vi "ReadWrite.ProcessData.vi"(8 "error in (no error)":errorcluster, 10 "timeout ms":i32=100, 11 "ReadWrite in":refnum<class "ReadWrite.lvclass">) -> (0 "error out":errorcluster, 1 "Timeout?":bool, 2 "Values":dbl[](array[numeric]), 3 "ReadWrite out":refnum<class "ReadWrite.lvclass">)   [LabVIEW 2015, in "Data Access Engine.lvlib" / "ReadWrite.lvclass"]
uses:
  ReadWrite.lvclass
  ReadWrite.lvclass/ReadWrite.ctl
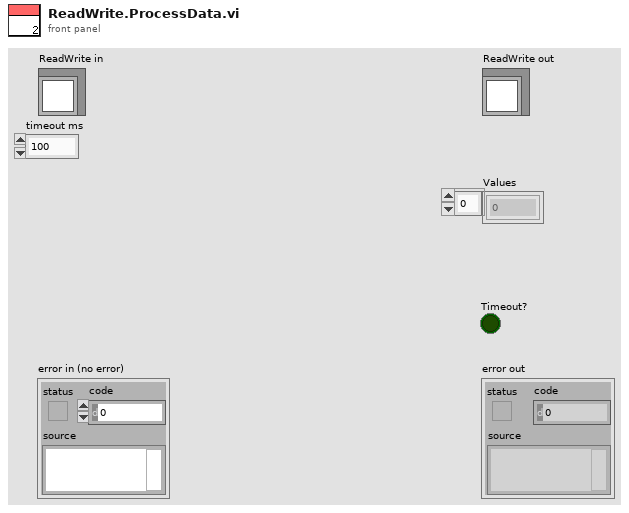
[diagram p1: front panel]
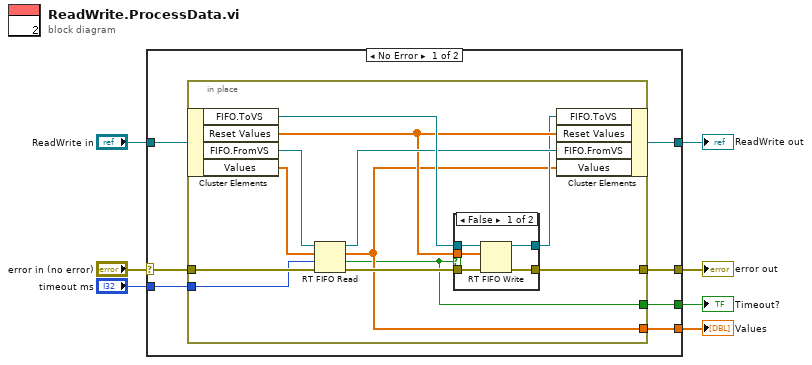
[diagram p0: block diagram]
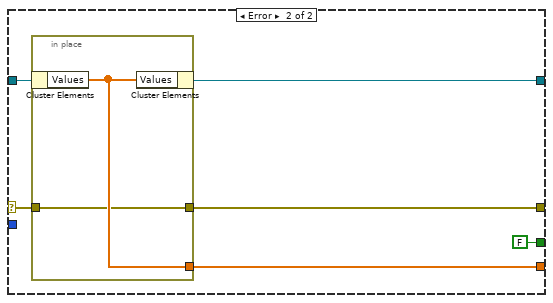
[diagram p3: hidden frame]
diagram:
  n1 = case shown="No Error" "error in (no error)" {
    selector: "error in (no error)" -> [w14 w35]
    tunnel: [w13 w36] -> w6
    tunnel: [w10 w38] -> w4
    tunnel: "ReadWrite in" -> [w11 w39]
    tunnel: [w12 w37] -> w3
    tunnel: "timeout ms" -> [w9 _]
    tunnel: [w8 FALSE ("empty?")] -> w1
    frame No Error {
      n2 = in-place {
        in-place-border: w14 -> [w25]
        in-place-border: [w18] -> w13
        in-place-border: [w17] -> w12
        in-place-border: w9 -> [w16]
        in-place-border: [w15] -> w8
        n3 = in-place-cluster #1(w11) -> ("FIFO.ToVS"=w22:refnum<k33>, "Reset Values"=w20:dbl[], "FIFO.FromVS"=w26:refnum<k33>, "Values"=w24:dbl[])
        n4 = RT FIFO Read(0:w26, 1:w24, 2:w16, 3:w25) -> (8:w21:refnum<k33>, 9:w17:dbl[], 10:w15:bool, 11:w23:errorcluster)  [unwired: 1 out]
        n5 = case shown="False" w15 {
          tunnel: w23 -> [w31 w32]
          tunnel: w20 -> [w30 _]
          tunnel: w22 -> [w29 w33]
          tunnel: [w28 w33] -> w19
          tunnel: [w27 w32] -> w18
          frame False {
            n6 = RT FIFO Write(0:w29, 1:w30, 3:w31) -> (8:w28:refnum<k33>, 11:w27:errorcluster)  [unwired: 2 in, 2 out]
          }
          frame True {
          }
        }
        n7 = in-place-cluster #1("FIFO.ToVS"=w19, "Reset Values"=w20, "FIFO.FromVS"=w21, "Values"=w17) -> (w10:refnum<class "ReadWrite.lvclass">)
      }
    }
    frame Error {
      n8 = in-place {
        in-place-border: [w41] -> w37
        in-place-border: [w40] -> w36
        in-place-border: w35 -> [w40]
        n9 = in-place-cluster #2(w39) -> ("Values"=w41:dbl[])
        n10 = in-place-cluster #2("Values"=w41) -> (w38:refnum<class "ReadWrite.lvclass">)
      }
    }
  }
  "error out" <- w6
  "ReadWrite out" <- w4
  "Values" <- w3
  "Timeout?" <- w1
